vi "Publish.vi"(4 "timeout (1000ms)":i32=1000, 6 "QoS":T1, 8 "error in (no error)":errorcluster, 9 "Payload":variant, 10 "Topic Name (empty: Payload name)":string, 11 "Client in":refnum<class "Client.lvclass">) -> (0 "error out":errorcluster, 2 "Published":bool, 3 "Client out":refnum<class "Client.lvclass">)   [LabVIEW 2013, in "MQTT Client.lvlib" / "Client.lvclass"]
uses:
  Client.lvclass
  <vilib>/LabVIEW Open Source Project/MQTT Control Packets/Control Packets/ControlPacket/QualityOfService -- enum.ctl
  MQTT_Base/Base Class/MQTT_Base.lvclass/MQTT_Base.ctl
  <vilib>/LabVIEW Open Source Project/MQTT Control Packets/Control Packets/PUBLISH/PUBLISH.lvclass
  <vilib>/LabVIEW Open Source Project/MQTT Control Packets/Control Packets/PUBCOMP/PUBCOMP.lvclass
  <vilib>/LabVIEW Open Source Project/MQTT Control Packets/Control Packets/PUBREC/PUBREC.lvclass
  <vilib>/LabVIEW Open Source Project/MQTT Control Packets/Control Packets/ControlPacket/ControlPacket.lvclass/ControlPacket.ctl
  <vilib>/LabVIEW Open Source Project/MQTT Control Packets/Control Packets/PUBACK/PUBACK.lvclass
  <vilib>/LabVIEW Open Source Project/Data Manipulation/TypeDescriptor/TypeDescriptor_GetName.vi
  <vilib>/LabVIEW Open Source Project/Data Manipulation/TypeDescriptor/TypeDescriptor_GetPString.vi
  <vilib>/LabVIEW Open Source Project/Serializer/Serializer/Serializer.lvclass
  <vilib>/LabVIEW Open Source Project/MQTT Control Packets/Control Packets/ControlPacket/ControlPacket.lvclass
  MQTT_Base/Base Class/MQTT_Base.lvclass
  <vilib>/LabVIEW Open Source Project/Data Manipulation/Variant/OpenVariant.lvlib
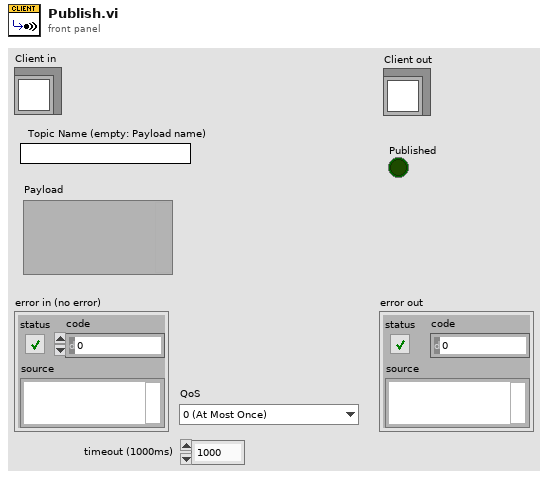
[diagram p1: front panel]
types:
  T1 = typedef "MQTT_Control_Packets.lvlib/ControlPacket.lvclass/QualityOfService -- enum.ctl" = enum16{"0 (At Most Once)", "1 (At Least Once)", "2 (Exactly Once)"}
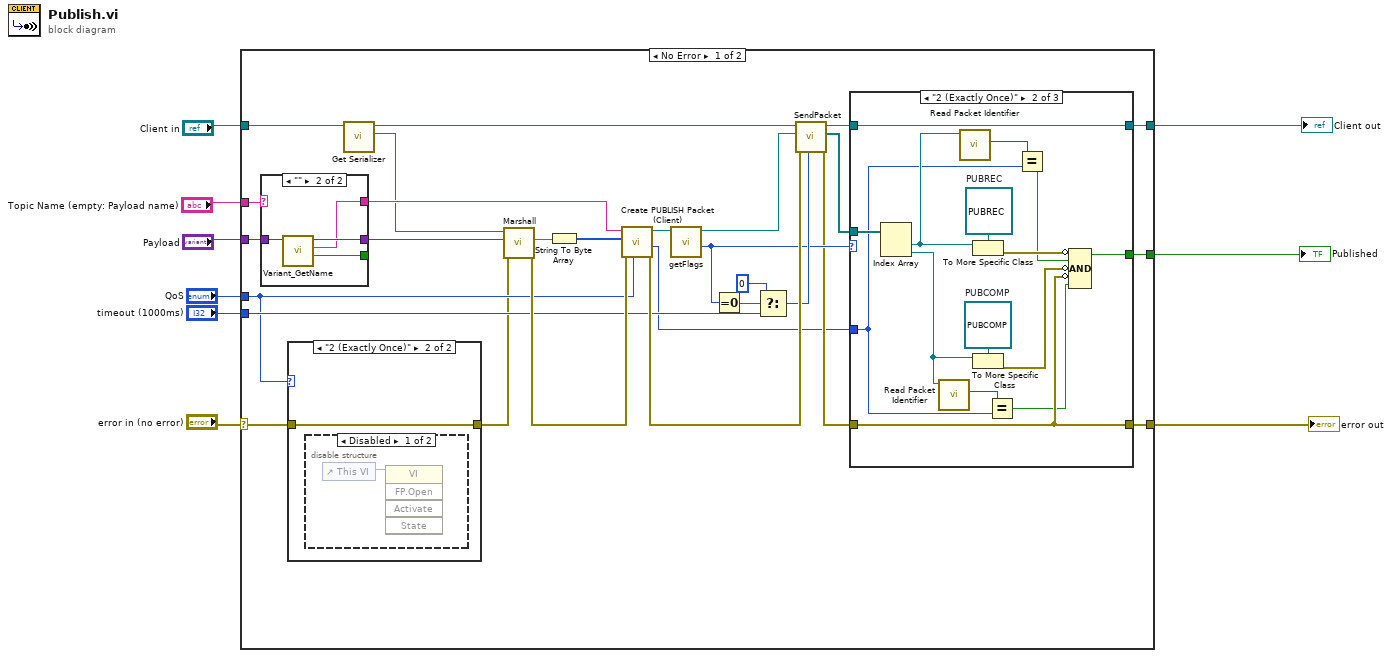
[diagram p0: block diagram]
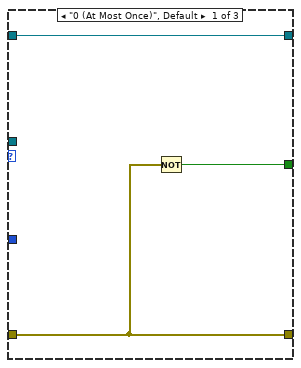
[diagram p4: hidden frame]
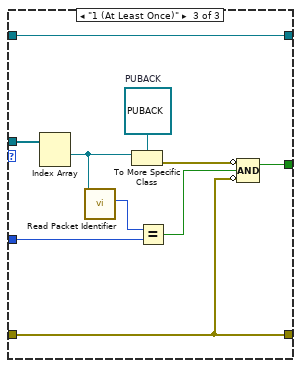
[diagram p5: hidden frame]
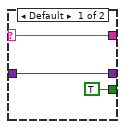
[diagram p6: hidden frame]
diagram:
  n1 = case shown="No Error" "error in (no error)" {
    selector: "error in (no error)" -> [w11 w77]
    tunnel: [w21 w77] -> w4
    tunnel: [w17 w76] -> w5
    tunnel: "Client in" -> [w15 w76]
    tunnel: "Payload" -> [w35 _]
    tunnel: "Topic Name (empty: Payload name)" -> [w33 _]
    tunnel: "QoS" -> [w12 _]
    tunnel: "timeout (1000ms)" -> [w24 _]
    tunnel: [w19 _] -> w1
    frame No Error {
      n2 = case shown="\"\"" w33 {
        selector: w33 -> [w71 _]
        tunnel: w35 -> [w70 w75]
        tunnel: [w70 w74] -> w34
        tunnel: [w71 w73] -> w32
        tunnel: [TRUE ("found") w72] -> _
        frame Default {
        }
        frame "" {
          n3 = call <vilib>:"Variant_GetName.vi"("Variant"=w75) -> ("found"=w72:bool, "Name"=w73:string, "Variant dup"=w74:variant)  [unwired: 8 in]
        }
      }
      n4 = case shown="\"2 (Exactly Once)\"" w12 {
        tunnel: [w38 w39] -> w10
        tunnel: w11 -> [w38 w39]
        frame Default {
        }
        frame "2 (Exactly Once)" {
          n5 = disable-structure shown="Disabled" {
            frame Disabled {
              n6 = control-ref of="This VI"() -> (w40:refnum<vi>)
              n7 = invoke class="VI" method="FP.Open"(reference=w40) -> ()  [unwired: 4 in, 5 out]
            }
            frame Enabled {
            }
          }
        }
      }
      n8 = call "Get Serializer.vi"("MQTT_Base"=w15) -> ("Serializer"=w13:refnum<class "Serializer.lvclass">, "MQTT_Base out"=w14:refnum<class "Client.lvclass">)  [unwired: 8 in, 1 out]
      n9 = call <vilib>:"Marshall.vi"("error in (no error)"=w10, "Variant"=w34, "Serializer in"=w13) -> ("error out"=w31:errorcluster, "String"=w37:string)  [unwired: 6 in, 1 out]
      n10 = String To Byte Array(string=w37) -> (unsigned byte array=w36:u8[])
      n11 = call <vilib>:"Create PUBLISH Packet (Client).vi"("QoS"=w12, "error in (no error)"=w31, "Payload"=w36, "Topic Name"=w32) -> ("error out"=w30:errorcluster, "Packet ID"=w16:u16, "PUBLISH"=w29:refnum<class "PUBLISH.lvclass">)  [unwired: 4 in, 1 out]
      n12 = call-dynamic "getFlags.vi"("PUBLISH in"=w29) -> ("QoS"=w22:T1, "PUBLISH out"=w28:refnum<class "PUBLISH.lvclass">)  [unwired: 7 in, 2 out]
      n13 = Equal To 0?(x=w22) -> (x = 0?=w26:bool)
      n14 = Select(t=0 ("timeout (0ms : no ack)"), s=w26, f=w24) -> (s? t:f=w23:i32)
      n15 = call "SendPacket.vi"("timeout (0ms : no ack)"=w23, "error in (no error)"=w30, "ControlPacket"=w28, "Client in"=w14) -> ("error out"=w20:errorcluster, "Response"=w27:refnum<class "ControlPacket.lvclass">[], "Client out"=w18:refnum<class "Client.lvclass">)  [unwired: 5 in]
      n16 = case shown="\"2 (Exactly Once)\"" w22 {
        tunnel: w27 -> [_ w58 w68]
        tunnel: [w43 w52 w63] -> w21
        tunnel: w20 -> [w43 w52 w63]
        tunnel: [w42 w53 w59] -> w19
        tunnel: w18 -> [w41 w49 w66]
        tunnel: [w41 w49 w66] -> w17
        tunnel: w16 -> [_ w44 w61]
        frame "0 (At Most Once)", Default {
          n17 = Not(x=w43) -> (.not. x?=w42:bool)
        }
        frame "2 (Exactly Once)" {
          w57 = refnum<class "PUBREC.lvclass"> refnum  # PUBREC
          w56 = refnum<class "PUBCOMP.lvclass"> refnum  # PUBCOMP
          n18 = Index Array(array=w58) -> (element #1=w47:refnum<class "ControlPacket.lvclass">, element #2=w46:refnum<class "ControlPacket.lvclass">)  [unwired: 2 in]
          n19 = call <vilib>:"Read Packet Identifier.vi"("ControlPacket in"=w46) -> ("Packet Identifier"=w51:u16)  [unwired: 9 in, 1 out]
          n20 = call <vilib>:"Read Packet Identifier.vi"("ControlPacket in"=w47) -> ("Packet Identifier"=w48:u16)  [unwired: 9 in, 1 out]
          n21 = To More Specific Class(target class=w57, reference=w47) -> (error out=w55:errorcluster)  [unwired: 1 in, 1 out]
          n22 = To More Specific Class(target class=w56, reference=w46) -> (error out=w54:errorcluster)  [unwired: 1 in, 1 out]
          n23 = Equal?(x=w51, y=w44) -> (x = y?=w50:bool)
          n24 = Equal?(x=w48, y=w44) -> (x = y?=w45:bool)
          n25 = Compound Arithmetic op=AND(invert w55, w45, invert w54, invert w52, w50) -> (w53:bool)
        }
        frame "1 (At Least Once)" {
          w67 = refnum<class "PUBACK.lvclass"> refnum  # PUBACK
          n26 = Index Array(array=w68) -> (element #1=w65:refnum<class "ControlPacket.lvclass">)  [unwired: 2 in, 1 out]
          n27 = call <vilib>:"Read Packet Identifier.vi"("ControlPacket in"=w65) -> ("Packet Identifier"=w62:u16)  [unwired: 9 in, 1 out]
          n28 = To More Specific Class(target class=w67, reference=w65) -> (error out=w64:errorcluster)  [unwired: 1 in, 1 out]
          n29 = Equal?(x=w62, y=w61) -> (x = y?=w60:bool)
          n30 = Compound Arithmetic op=AND(invert w64, w60, invert w63) -> (w59:bool)
        }
      }
    }
    frame Error {
    }
  }
  "error out" <- w4
  "Client out" <- w5
  "Published" <- w1
